vi "ReferencesGlobal.vi"(10 "Set?":bool, 11 "AscriptRefsIn":T1) -> (3 "AscriptRefsOut":T1)   [LabVIEW 2016]
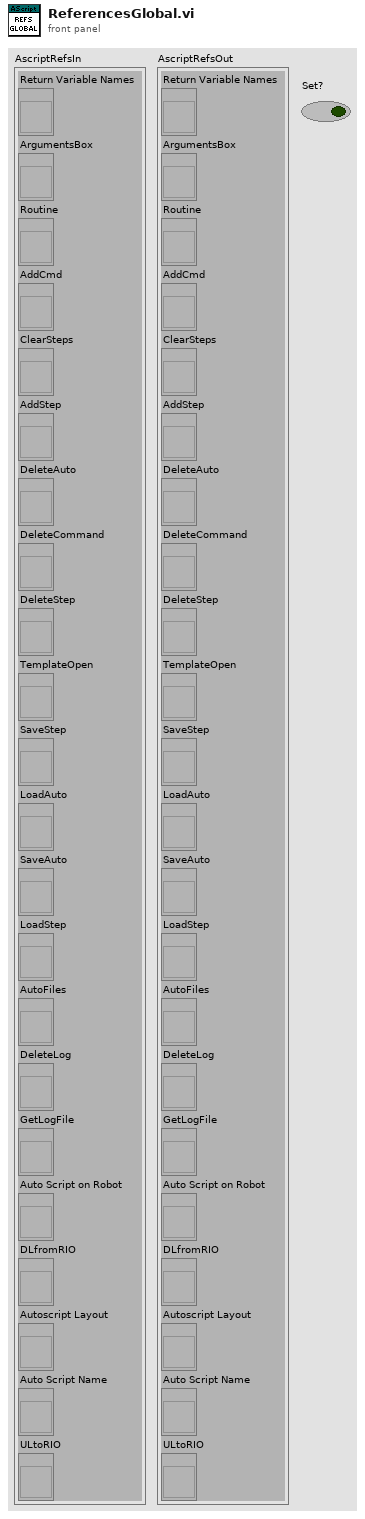
[diagram p1: front panel]
types:
  T1 = cluster{"Return Variable Names":refnum<vi>, "ArgumentsBox":refnum<vi>, "Routine":refnum<vi>, "AddCmd":refnum<vi>, "ClearSteps":refnum<vi>, "AddStep":refnum<vi>, "DeleteAuto":refnum<vi>, "DeleteCommand":refnum<vi>, "DeleteStep":refnum<vi>, "TemplateOpen":refnum<vi>, "SaveStep":refnum<vi>, "LoadAuto":refnum<vi>, "SaveAuto":refnum<vi>, "LoadStep":refnum<vi>, "AutoFiles":refnum<vi>, "DeleteLog":refnum<vi>, "GetLogFile":refnum<vi>, "Auto Script on Robot":refnum<vi>, "DLfromRIO":refnum<vi>, "Autoscript Layout":refnum<vi>, "Auto Script Name":refnum<vi>, "ULtoRIO":refnum<vi>}
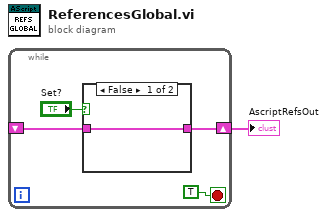
[diagram p0: block diagram]
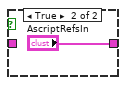
[diagram p2: hidden frame]
diagram:
  n1 = while {
    shift-right: [w3] -> w1
    shift-left: _ -> [w2]
    stop <- TRUE stop-if-true
    n2 = case shown="False" "Set?" {
      tunnel: [w6 "AscriptRefsIn"] -> w3
      tunnel: w2 -> [w6 _]
      frame False {
      }
      frame True {
      }
    }
  }
  "AscriptRefsOut" <- w1
